vi "UIDisable.vi"(8 "error in (no error)":errorcluster, 10 "UI":T1, 11 "Status:":refnum<vi>) -> (0 "error out":errorcluster)   [LabVIEW 2018]
uses:
  Global Variables.vi
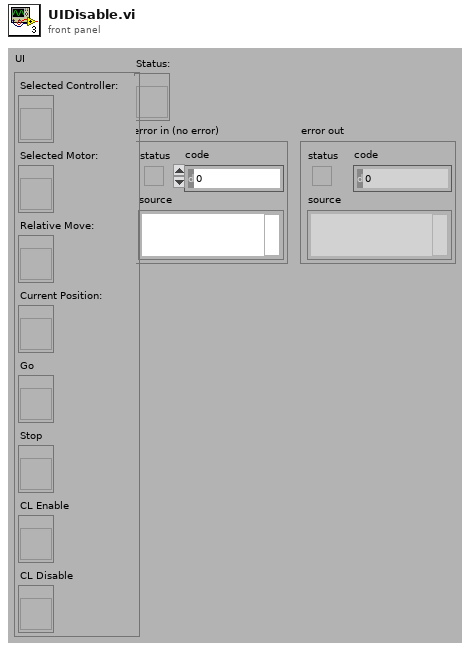
[diagram p1: front panel]
types:
  T1 = cluster{"Selected Controller:":refnum<vi>, "Selected Motor:":refnum<vi>, "Relative Move:":refnum<vi>, "Current Position:":refnum<vi>, "Go":refnum<vi>, "Stop":refnum<vi>, "CL Enable":refnum<vi>, "CL Disable":refnum<vi>}
  T2 = enum8{"Enabled", "Disabled", "Disabled and Grayed Out"}
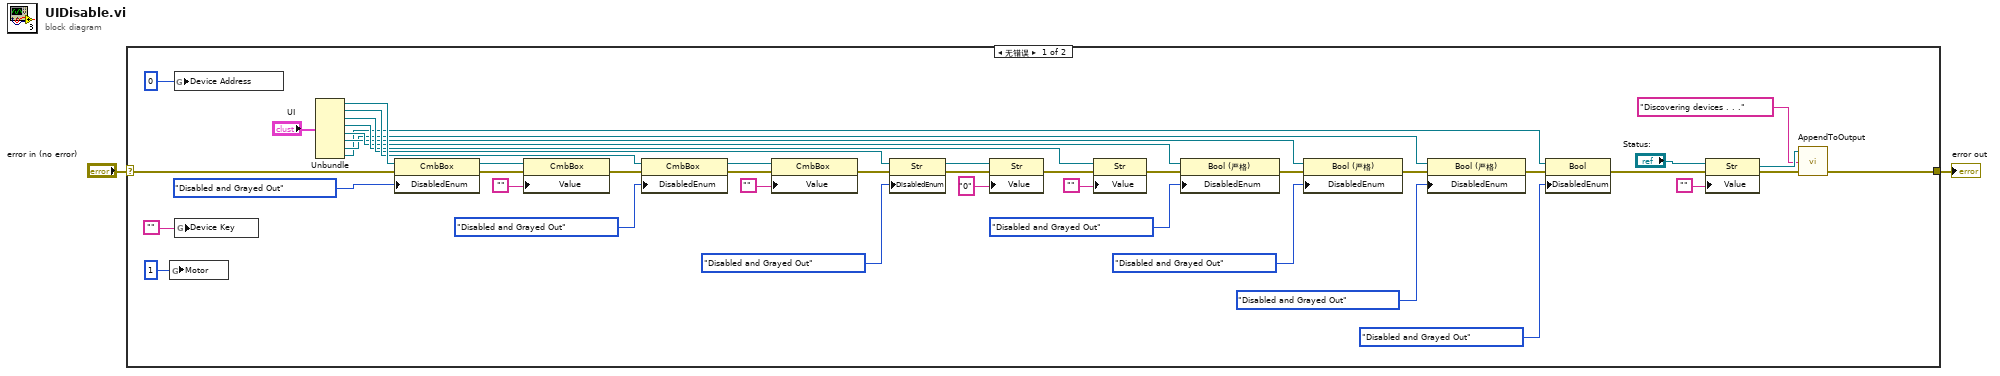
[diagram p0: block diagram]
diagram:
  n1 = case shown="无错误" "error in (no error)" {
    selector: "error in (no error)" -> [w37 w47]
    tunnel: [w27 w47] -> w1
    frame No Error {
      n2 = global write "Global Variables.vi" "Motor"(1 ("Motor")) -> ()
      n3 = global write "Global Variables.vi" "Device Address"(0 ("Device Address")) -> ()
      n4 = global write "Global Variables.vi" "Device Key"("") -> ()
      n5 = Unbundle("UI") -> ("Selected Controller:"=w13:refnum<vi>, "Selected Motor:"=w12:refnum<vi>, "Relative Move:"=w11:refnum<vi>, "Current Position:"=w10:refnum<vi>, "Go"=w9:refnum<vi>, "Stop"=w8:refnum<vi>, "CL Enable"=w7:refnum<vi>, "CL Disable"=w3:refnum<vi>)
      n6 = property on="Property Node" class="CmbBox"(reference=w13, error in=w37, "DisabledEnum"=T2."Disabled and Grayed Out" ("Disabled")) -> (reference out=w36:refnum<vi>, error out=w32:errorcluster)
      n7 = property class="CmbBox"(reference=w36, error in=w32, "Value"="") -> (error out=w31:errorcluster)  [unwired: 1 out]
      n8 = property on="Property Node" class="CmbBox"(reference=w12, error in=w31, "DisabledEnum"=T2."Disabled and Grayed Out" ("Disabled")) -> (reference out=w34:refnum<vi>, error out=w30:errorcluster)
      n9 = property class="CmbBox"(reference=w34, error in=w30, "Value"="") -> (error out=w29:errorcluster)  [unwired: 1 out]
      n10 = property on="Property Node" class="Str"(reference=w11, error in=w29, "DisabledEnum"=T2."Disabled and Grayed Out" ("Disabled")) -> (reference out=w21:refnum<vi>, error out=w22:errorcluster)
      n11 = property class="Str"(reference=w21, error in=w22, "Value"="0") -> (error out=w19:errorcluster)  [unwired: 1 out]
      n12 = property on="Property Node" class="Str"(reference=w10, error in=w19, "Value"="") -> (error out=w18:errorcluster)  [unwired: 1 out]
      n13 = property on="Property Node" class="Bool (严格)"(reference=w9, error in=w18, "DisabledEnum"=T2."Disabled and Grayed Out" ("Disabled")) -> (error out=w40:errorcluster)  [unwired: 1 out]
      n14 = property on="Property Node" class="Bool (严格)"(reference=w8, error in=w40, "DisabledEnum"=T2."Disabled and Grayed Out" ("Disabled")) -> (error out=w39:errorcluster)  [unwired: 1 out]
      n15 = property on="Property Node" class="Bool (严格)"(reference=w7, error in=w39, "DisabledEnum"=T2."Disabled and Grayed Out" ("Disabled")) -> (error out=w4:errorcluster)  [unwired: 1 out]
      n16 = property on="Property Node" class="Bool"(reference=w3, error in=w4, "DisabledEnum"=T2."Disabled and Grayed Out" ("Disabled")) -> (error out=w5:errorcluster)  [unwired: 1 out]
      n17 = property class="Str"(reference="Status:", error in=w5, "Value"="") -> (reference out=w28:refnum<vi>, error out=w26:errorcluster)
      n18 = call "AppendToOutput.vi"("error in"=w26, "Input String"="Discovering devices . . .", "Output Refnum In"=w28) -> ("error out"=w27:errorcluster)  [unwired: 1 in, 1 out]
    }
    frame Error {
    }
  }
  "error out" <- w1
